vi "DynamicChannelMapping Value Change.vi"(7 "Control Refs":T1, 9 "Enable Dynamic Mapping":bool, 10 "Channel Subscription Pattern Matches":string[](array[string]), 11 "References":T2) -> (0 "error out":errorcluster)   [LabVIEW 2015, in "TDMS datalogger editor node.lvclass"]
uses:
  TDMS datalogger editor node.lvclass
  <vilib>/NI/DCAF/Tag Editor Core/Table API/Table Manager/object ref.ctl
  <vilib>/NI/DCAF/Tag Editor Core/Configuration Editor/Classes/Engine Parent/Engine Parent Editor Node.lvclass
  <vilib>/NI/DCAF/Tag Editor Core/Configuration Editor/Classes/Module editor node/module editor node.lvclass
  Control Refs.ctl
  TDMS datalogger editor node.lvclass/TDMS datalogger editor node.ctl
  module/configuration/TDMS datalogger configuration.lvclass/TDMS datalogger configuration.ctl
  module/configuration/Write channel pattern matches.vi
  module/configuration/TDMS datalogger configuration.lvclass
  <vilib>/NI/DCAF/Tag Editor Core/Table API/Table Manager/Table Manager.lvclass
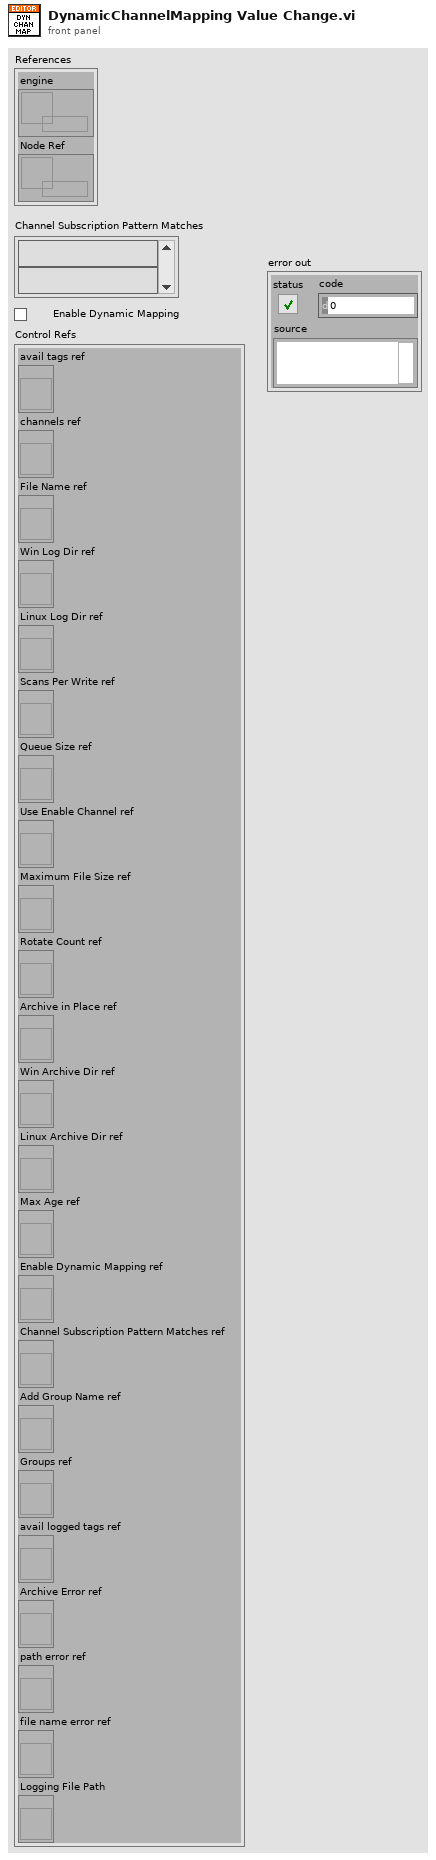
[diagram p1: front panel]
types:
  T1 = typedef "Control Refs.ctl" = cluster{"avail tags ref":refnum<vi>, "channels ref":refnum<vi>, "File Name ref":refnum<vi>, "Win Log Dir ref":refnum<vi>, "Linux Log Dir ref":refnum<vi>, "Scans Per Write ref":refnum<vi>, "Queue Size ref":refnum<vi>, "Use Enable Channel ref":refnum<vi>, "Maximum File Size ref":refnum<vi>, "Rotate Count ref":refnum<vi>, "Archive in Place ref":refnum<vi>, "Win Archive Dir ref":refnum<vi>, "Linux Archive Dir ref":refnum<vi>, "Max Age ref":refnum<vi>, "Enable Dynamic Mapping ref":refnum<vi>, "Channel Subscription Pattern Matches ref":refnum<vi>, "Add Group Name ref":refnum<vi>, "Groups ref":refnum<vi>, "avail logged tags ref":refnum<vi>, "Archive Error ref":refnum<vi>, "path error ref":refnum<vi>, "file name error ref":refnum<vi>, "Logging File Path":refnum<vi>}
  T2 = typedef "Table Manager.lvlib/Table Manager.lvclass/object ref.ctl" = cluster{"engine":refnum<data-value>, "Node Ref":refnum<data-value>}
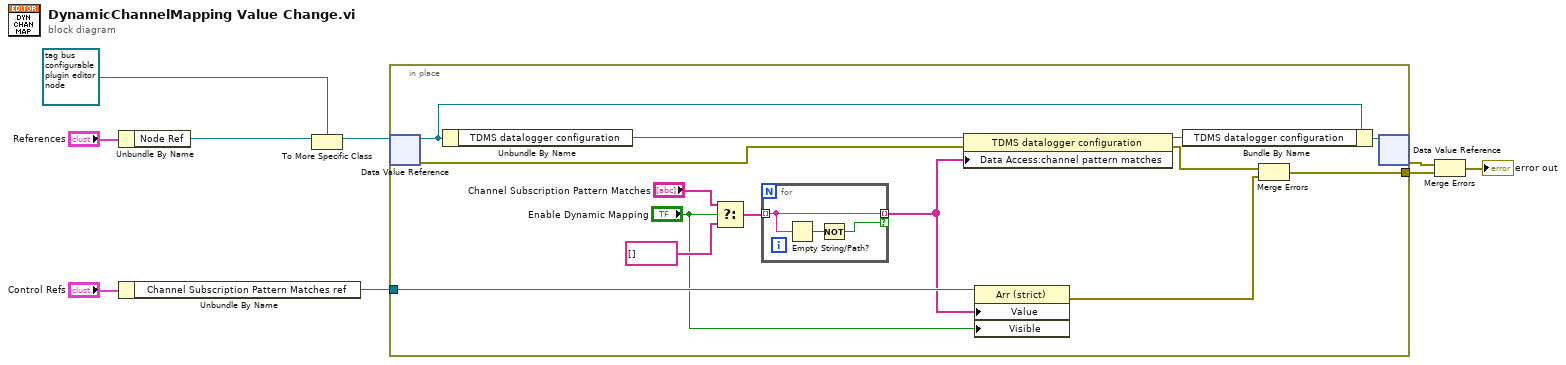
[diagram p0: block diagram]
diagram:
  n1 = Unbundle By Name("References") -> ("Node Ref"=w8:refnum<data-value>)
  n2 = Unbundle By Name("Control Refs") -> ("Channel Subscription Pattern Matches ref"=w1:refnum<vi>)
  n3 = To More Specific Class(target class=refnum<data-value> refnum ("data value reference"), reference=w8) -> (specific class reference=w6:refnum<data-value>)  [unwired: 1 in, 1 out]
  n4 = in-place {
    in-place-border: [w14] -> w5
    in-place-border: w1 -> [w12]
    n5 = in-place-dvr #1(w6) -> (w22:refnum<class "TDMS datalogger editor node.lvclass">, w16:errorcluster)
    n6 = Unbundle By Name(w22) -> ("TDMS datalogger configuration"=w17:refnum<class "TDMS datalogger configuration.lvclass">)
    n7 = Select(t="Channel Subscription Pattern Matches", s="Enable Dynamic Mapping", f=string[] []) -> (s? t:f=w19:string[])
    n8 = for {
      tunnel: w19 -> [w26] mode=indexing
      tunnel: [w26] -> w10 mode=indexing if=w24
      n9 = Empty String/Path?(string/path=w26) -> (empty?=w25:bool)
      n10 = Not(x=w25) -> (.not. x?=w24:bool)
    }
    n11 = property class="TDMS datalogger configuration"(reference=w17, error in=w16, "Data Access:channel pattern matches"=w10) -> (reference out=w18:refnum<class "TDMS datalogger configuration.lvclass">, error out=w15:errorcluster)
    n12 = property on="Property Node" class="Arr (strict)"(reference=w12, "Value"=w10, "Visible"="Enable Dynamic Mapping") -> (error out=w13:errorcluster)  [unwired: 1 in, 1 out]
    n13 = Bundle By Name(cluster=w22, "TDMS datalogger configuration"=w18) -> (w23:refnum<class "TDMS datalogger editor node.lvclass">)
    n14 = Merge Errors(w15, w13) -> (w14:errorcluster)
    n15 = in-place-dvr #1(w23) -> (w3:errorcluster)  [unwired: 1 out]
  }
  n16 = Merge Errors(w3, w5) -> (→"error out":errorcluster)
